vi "potential-field - Copia.vi"(11 "IA State Output in":T1={"our_robots"=[], "enemy_robots"=[], "balls"=[], "geometry"={"line_width"=0, "field_length"=0, "field_width"=0, "boundary_width"=0, "referee_width"=0, "goal_width"=0, "goal_depth"=0, "goal_wall_width"=0, "center_circle_radius"=0, "defense_radius"=0, "defense_stretch"=0, "free_kick_from_defense_dist"=0, "penalty_spot_from_field_line_dist"=0, "penalty_line_from_spot_dist"=0}, "IA Judge"={"stage"="", "command"="", "our_goalie_id"=0.0, "enemy_goalie_id"=0.0, "command\nenum"=enum."Halt", "Time"=enum."Azul"}, "Received Timestamp"=timestamp(0 s since 1904-01-01), "Events"={"Touch"=FALSE, "Ball out"=FALSE, "id touch"=0.0, "Ball out of \nVision"=FALSE, "Ball inside \nGoalie area"=FALSE, "Robot not responding"=FALSE, "Robots responding status"=[1.0, 1.0, 1.0, 1.0, 1.0, 1.0]}}) -> (3 "IA State Output out":T1={"our_robots"=[], "enemy_robots"=[], "balls"=[], "geometry"={"line_width"=0, "field_length"=0, "field_width"=0, "boundary_width"=0, "referee_width"=0, "goal_width"=0, "goal_depth"=0, "goal_wall_width"=0, "center_circle_radius"=0, "defense_radius"=0, "defense_stretch"=0, "free_kick_from_defense_dist"=0, "penalty_spot_from_field_line_dist"=0, "penalty_line_from_spot_dist"=0}, "IA Judge"={"stage"="", "command"="", "our_goalie_id"=0.0, "enemy_goalie_id"=0.0, "command\nenum"=enum."Halt", "Time"=enum."Azul"}, "Received Timestamp"=timestamp(0 s since 1904-01-01), "Events"={"Touch"=FALSE, "Ball out"=FALSE, "id touch"=0.0, "Ball out of \nVision"=FALSE, "Ball inside \nGoalie area"=FALSE, "Robot not responding"=FALSE, "Robots responding status"=[1.0, 1.0, 1.0, 1.0, 1.0, 1.0]}})   [LabVIEW 2016]
uses:
  Core/AI Input.ctl
  Core/AI Robot.ctl
  Intel/Functions Enum.ctl
  Core/AI Ball.ctl
  Core/Field Size.ctl
  Core/AI Judge.ctl
  Intel/Command Enum.ctl
  <vilib>/Analysis/_algsub.llb/Real Vector Norm.vi
  <vilib>/Analysis/coordinate.llb/2D Cartesian Coordinate Rotation (Scalar).vi
  <vilib>/Analysis/NI_AALPro.lvlib
panel:
  in  "dist to nullify":dbl
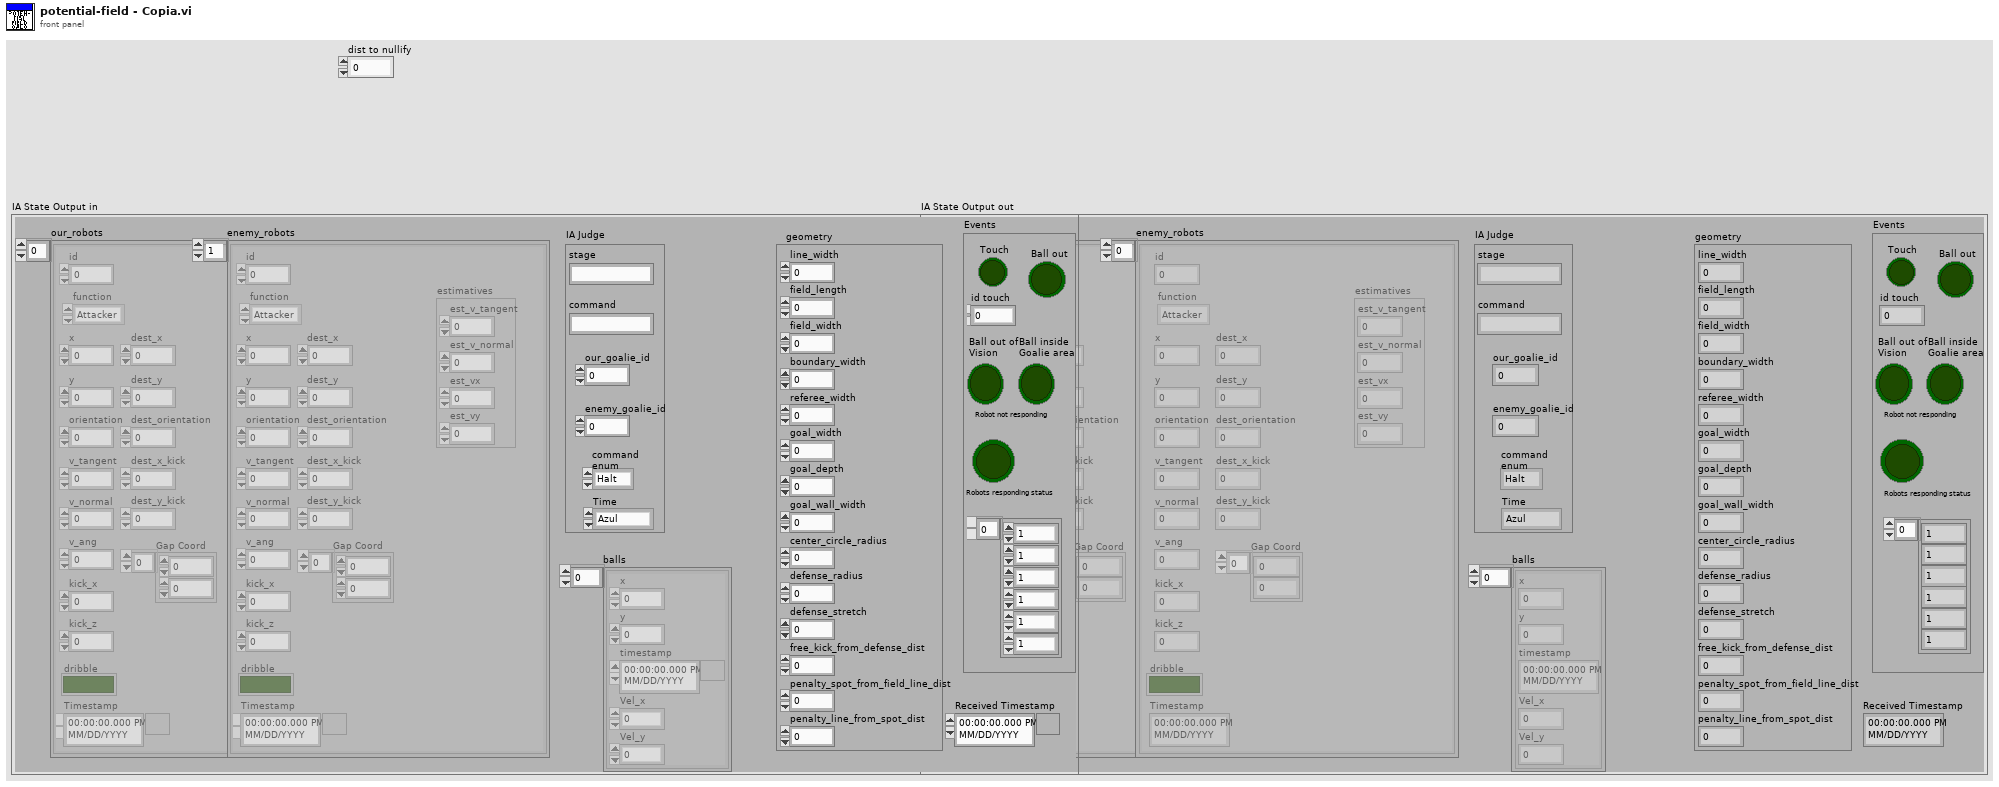
[diagram p1: front panel]
types:
  T1 = typedef "AI Input.ctl" = cluster{"our_robots":T2[], "enemy_robots":T2[], "balls":T4[], "geometry":T5, "IA Judge":T6, "Received Timestamp":timestamp, "Events":cluster{"Touch":bool, "Ball out":bool, "id touch":dbl, "Ball out of \nVision":bool, "Ball inside \nGoalie area":bool, "Robot not responding":bool, "Robots responding status":dbl[]}}
  T2 = typedef "AI Robot.ctl" = cluster{"id":u32, "function":T3, "x":dbl, "y":dbl, "orientation":dbl, "v_tangent":dbl, "v_normal":dbl, "v_ang":dbl, "kick_x":dbl, "kick_z":dbl, "dribble":bool, "Timestamp":timestamp, "dest_x":dbl, "dest_y":dbl, "dest_orientation":dbl, "estimatives":cluster{"est_v_tangent":dbl, "est_v_normal":dbl, "est_vx":dbl, "est_vy":dbl}, "dest_x_kick":dbl, "dest_y_kick":dbl, "Gap Coord":dbl[]}
  T3 = typedef "Functions Enum.ctl" = enum16{"Attacker", "Goalie", "Defender", "Striker", "Goto 0", "Dummy", "ZigZag"}
  T4 = typedef "AI Ball.ctl" = cluster{"x":dbl, "y":dbl, "timestamp":timestamp, "Vel_x":dbl, "Vel_y":dbl}
  T5 = typedef "Field Size.ctl" = cluster{"line_width":u32, "field_length":u32, "field_width":u32, "boundary_width":u32, "referee_width":u32, "goal_width":u32, "goal_depth":u32, "goal_wall_width":u32, "center_circle_radius":u32, "defense_radius":u32, "defense_stretch":u32, "free_kick_from_defense_dist":u32, "penalty_spot_from_field_line_dist":u32, "penalty_line_from_spot_dist":u32}
  T6 = typedef "AI Judge.ctl" = cluster{"stage":string, "command":string, "our_goalie_id":dbl, "enemy_goalie_id":dbl, "command\nenum":T7, "Time":enum16{"Azul", "Amarelo"}}
  T7 = typedef "Command Enum.ctl" = enum16{"Halt", "Stop", "Force Start", "PKA Normal Start", "Prepare Kickoff Ally", "PKE Normal Start", "Prepare Kickoff Enemy", "Prepare Penalty Ally", "PPA Normal Start", "Prepare Penalty Enemy", "PPE Normal Start", "Direct Free Enemy", "Direct Free Ally", "Indirect Free Enemy", "Indirect Free Ally", "Timeout Enemy", "Timeout Ally", "Goal Enemy", "Goal Ally", "Ball Placement Enemy", "Ball Placement Ally", "None"}
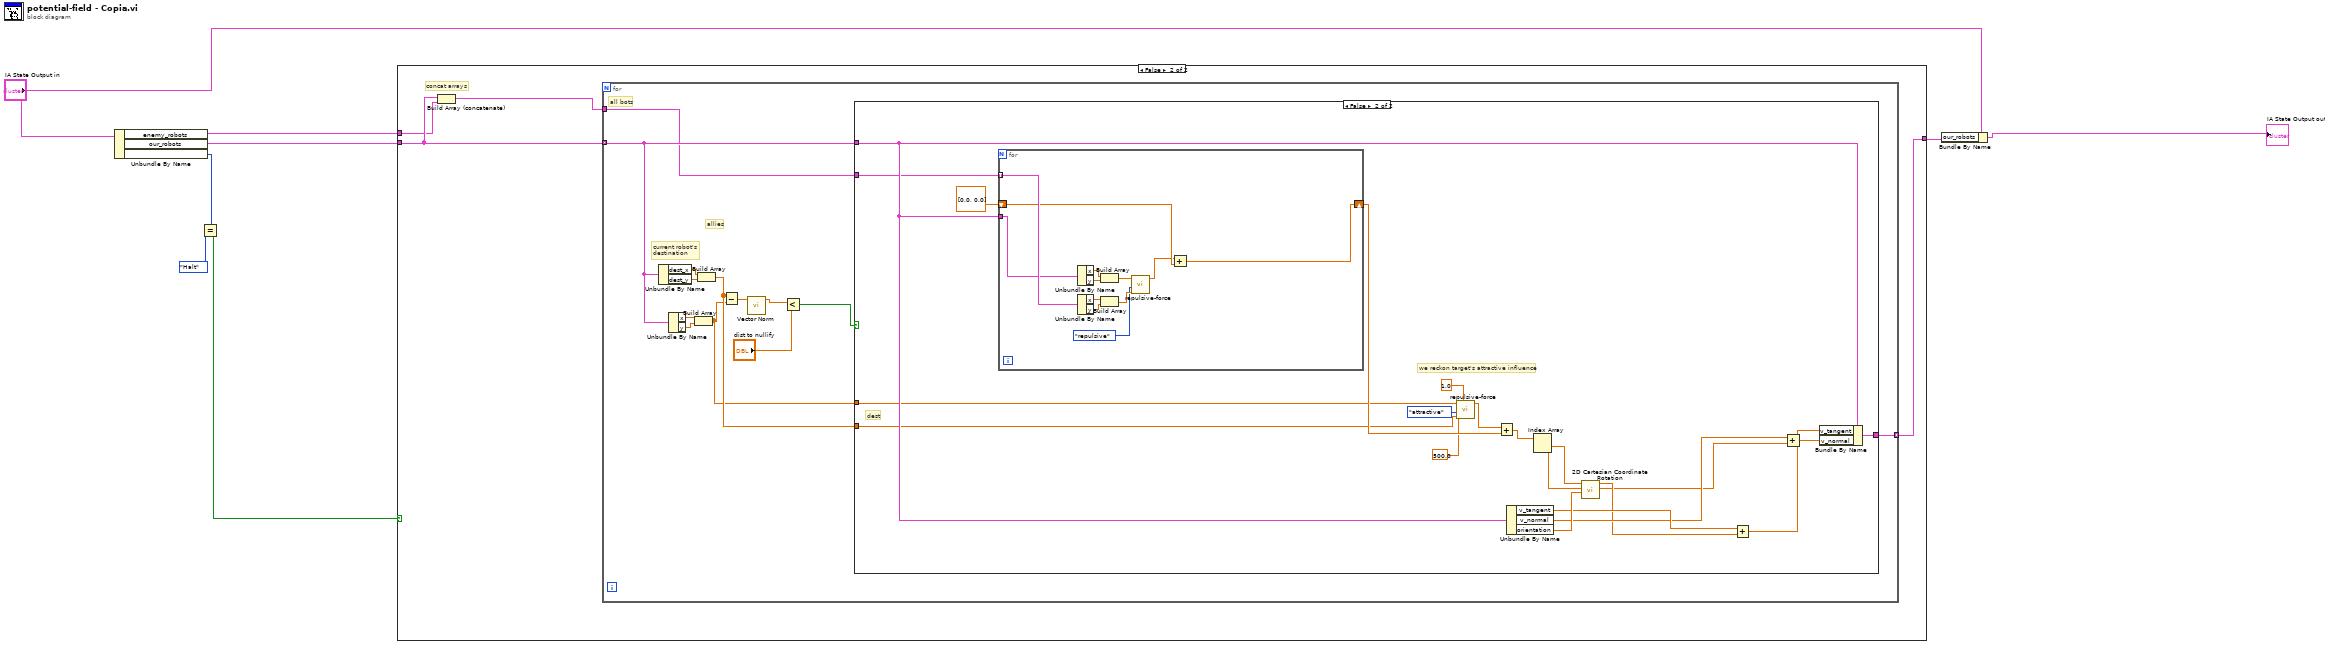
[diagram p0: block diagram]
diagram:
  n1 = Unbundle By Name("IA State Output in") -> ("enemy_robots"=w8:T2[], "our_robots"=w7:T2[], "IA Judge.command\nenum"=w2:T7)
  n2 = Equal?(x=w2, y=Command_Enum."Halt") -> (x = y?=w1:bool)
  n3 = case shown="False" w1 {
    tunnel: w8 -> [_ w12]
    tunnel: w7 -> [w9 w13]
    tunnel: [w9 w10] -> w6
    frame True {
    }
    frame False {
      # "concat arrays"
      n4 = Build Array (concatenate)(w13, w12) -> (w11:T2[])
      n5 = for {
        tunnel: w13 -> [w23] mode=indexing
        tunnel: [w26] -> w10 mode=indexing
        tunnel: w11 -> [w19]
        # "all bots"
        # "current robot's\ndestination"
        # "allies"
        n6 = Unbundle By Name(w23) -> ("dest_x"=w24:dbl, "dest_y"=w25:dbl)
        n7 = Unbundle By Name(w23) -> ("x"=w22:dbl, "y"=w21:dbl)
        n8 = Build Array(w22, w21) -> (w14:dbl[])
        n9 = Build Array(w24, w25) -> (w15:dbl[])
        n10 = Subtract(x=w15, y=w14) -> (x-y=w20:dbl[])
        n11 = call-poly <vilib>:"Vector Norm.vi"("Input Vector"=w20) -> ("norm"=w18:dbl)  [unwired: 9 in, 1 out]
        n12 = Less?(x=w18, y="dist to nullify") -> (x < y?=w16:bool)
        n13 = case shown="False" w16 {
          tunnel: [w27 w39] -> w26
          tunnel: w23 -> [w27 w37]
          tunnel: w19 -> [_ w36]
          tunnel: w15 -> [_ w34]
          tunnel: w14 -> [_ w33]
          frame True {
          }
          frame False {
            # "we reckon target's attractive influence"
            # "dest"
            n14 = for {
              tunnel: w36 -> [w60] mode=indexing
              tunnel: w37 -> [w53]
              shift-right: [w54] -> w35
              shift-left: dbl[] [0.0, 0.0] -> [w55]
              n15 = Unbundle By Name(w53) -> ("x"=w57:dbl, "y"=w56:dbl)
              n16 = Unbundle By Name(w60) -> ("x"=w59:dbl, "y"=w58:dbl)
              n17 = Build Array(w57, w56) -> (w52:dbl[])
              n18 = Build Array(w59, w58) -> (w51:dbl[])
              n19 = call "repulsive-force.vi"("obstacle pos"=w51, "force-type"=enum16{"repulsive", "attractive"}."repulsive", "agent pos"=w52) -> ("force"=w50:dbl[])  [unwired: 7 in, 1 out]
              n20 = Add(x=w50, y=w55) -> (x+y=w54:dbl[])
            }
            n21 = call "repulsive-force.vi"("max dist (greater)"=500.0, "multiplier"=1.0, "obstacle pos"=w34, "force-type"=enum16{"repulsive", "attractive"}."attractive", "agent pos"=w33) -> ("force"=w29:dbl[])  [unwired: 5 in, 1 out]
            n22 = Add(x=w29, y=w35) -> (x+y=w28:dbl[])
            n23 = Unbundle By Name(w37) -> ("v_tangent"=w45:dbl, "v_normal"=w44:dbl, "orientation"=w46:dbl)
            n24 = Index Array(array=w28) -> (element #1=w48:dbl, element #2=w47:dbl)  [unwired: 2 in]
            n25 = call-poly <vilib>:"2D Cartesian Coordinate Rotation.vi"("theta"=w46, "y"=w47, "x"=w48) -> ("y out"=w42:dbl, "x out"=w43:dbl)  [unwired: 6 in, 1 out]
            n26 = Add(x=w45, y=w43) -> (x+y=w41:dbl)
            n27 = Add(x=w44, y=w42) -> (x+y=w40:dbl)
            n28 = Bundle By Name(cluster=w37, "v_tangent"=w41, "v_normal"=w40) -> (w39:T2)
          }
        }
      }
    }
  }
  n29 = Bundle By Name(cluster="IA State Output in", "our_robots"=w6) -> (→"IA State Output out":T1)
